vi "LV SciSDK INIT RATEMETER.vi"(3 "error in (no error)":errorcluster, 4 "Board Handle In":T1, 5 "Ratemeter Name":string) -> (0 "error out":errorcluster, 1 "Board Handle Out":T1, 2 "Digitizer Handle Out":T2)   [LabVIEW 2021, in "SciSDK_Labview.lvlib"]
uses:
  SciSDK_Labview.lvlib
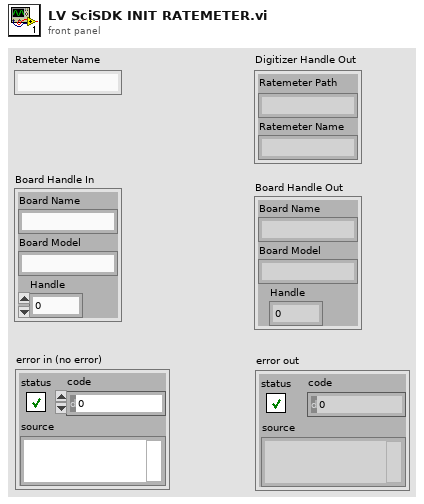
[diagram p1: front panel]
types:
  T1 = cluster{"Board Name":string, "Board Model":string, "Handle":u64}
  T2 = cluster{"Ratemeter Path":string, "Ratemeter Name":string}
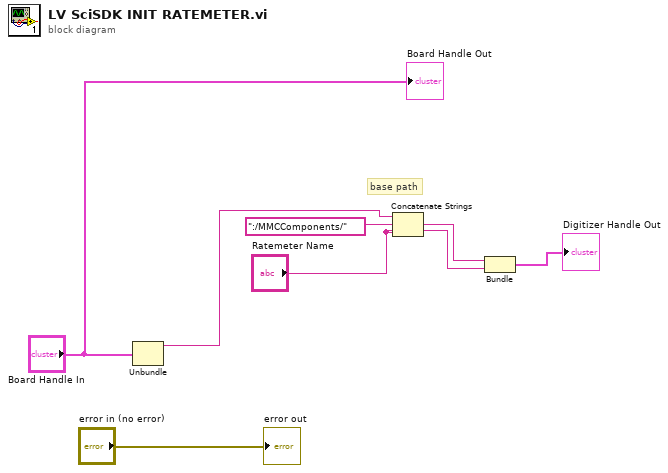
[diagram p0: block diagram]
diagram:
  # "base path"
  n1 = Unbundle("Board Handle In") -> ("Board Name"=w6:string)  [unwired: 2 out]
  n2 = Concatenate Strings(w6, ":/MMCComponents/" ("string"), "Ratemeter Name") -> (w5:string)
  n3 = Bundle(w5, "Ratemeter Name"="Ratemeter Name") -> (→"Digitizer Handle Out":cluster{string, "Ratemeter Name":string})  [unwired: 1 in]
  "error out" <- "error in (no error)"
  "Board Handle Out" <- "Board Handle In"
